vi "onDependencyConfigChanged.vi"(4 "Source GUID":string, 6 "keys changed":string[](array[string]), 8 "error in":errorcluster, 9 "Dependency":refnum<class "SMO.lvclass">, 11 "SMO in":refnum<class "SMO.lvclass">) -> (0 "error out":errorcluster, 3 "SMO out":refnum<class "SMO.lvclass">)   [LabVIEW 2021, in "smo.lvlib" / "SMO.lvclass"]
uses:
  SMO.lvclass
  SMO.lvclass/SMO.ctl
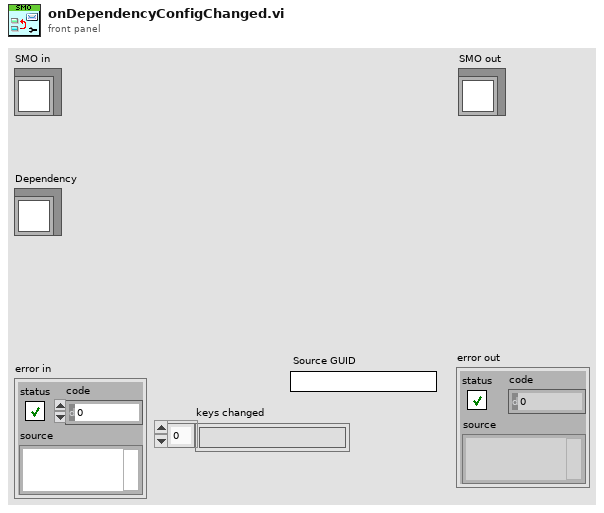
[diagram p1: front panel]
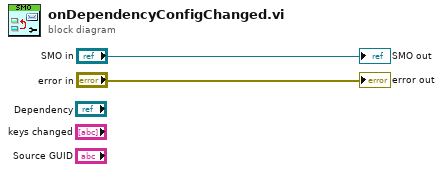
[diagram p0: block diagram]
diagram:
  "SMO out" <- "SMO in"
  "error out" <- "error in"
